vi "CH_LM App History.vi"(0 "Data":T1[](array[typedef]) {"Histogram"."X Values" format="%0.2f"; "Statistics"."Std. Dev." format="%#_4p"; "Statistics"."Max" format="%#_4p"; "Statistics"."Min" format="%#_4p"; "Statistics"."Mean" format="%#_4p"; "Data Cluster"."Flags" format="%.0b"; "Data Cluster"."Unit ID" format="%.0b"; "Data Cluster"."Quad Distance"."Y" format="%#.1f"; "Data Cluster"."Quad Distance"."X" format="%#.1f"; "Data Cluster"."Value" format="%#.7e"; "LabMax Device List Element"."Probe Diameter" format="%#.2g"}, 1 "Point(s)":i32, 2 "Sample Collection":enum32{"Fixed", "Continuous"}(ring), 3 "Sample Size":i32, 5 "Samples":i32, 7 "Point(s) Array":u32[](array[numeric]) min=1 max=20000, 9 "Points":i32, 11 "History in":T4[](array[typedef]) {"Stat. Min." format="%^#_7e"; "Stat. Max." format="%^#_7e"; "Maximum" format="%^#_7e"; "Live" format="%^#_7e"; "Value" format="%^#_7e"}, 12 "NofBins":i32, 13 "initialize Stat":bool, 14 "init Live Array":bool[](array[boolean])) -> (4 "Trend Data":T1[](array[typedef]) {"Histogram"."X Values" format="%0.2f"; "Statistics"."Std. Dev." format="%#_4p"; "Statistics"."Max" format="%#_4p"; "Statistics"."Min" format="%#_4p"; "Statistics"."Mean" format="%#_4p"; "Data Cluster"."Flags" format="%.0b"; "Data Cluster"."Unit ID" format="%.0b"; "Data Cluster"."Quad Distance"."Y" format="%#.1f"; "Data Cluster"."Quad Distance"."X" format="%#.1f"; "Data Cluster"."Value" format="%#.7e"; "LabMax Device List Element"."Probe Diameter" format="%#.2g"}, 15 "History out":T4[](array[typedef]) {"Stat. Min." format="%^#_7e"; "Stat. Max." format="%^#_7e"; "Maximum" format="%^#_7e"; "Live" format="%^#_7e"; "Value" format="%^#_7e"})   [LabVIEW 2012, in "CH_LM App.lvlib"]
doc: "This VI is used to calculate staticical properties, histogram data and to update the history data arrays."
uses:
  CH_LM App.lvlib
  <vilib>/Analysis/NI_AALBase.lvlib
  <vilib>/ptbypt/NI_PtbyPt.lvlib
  <vilib>/Analysis/baseanly.llb/Mean (DBL).vi
  CH_LM App DeviceListElement.ctl
  CH_LM/CH_LM Streaming Data.ctl
  CH_LM.lvlib
  CH_LM App TrendingData.ctl
  CH_LM App HistoryData.ctl
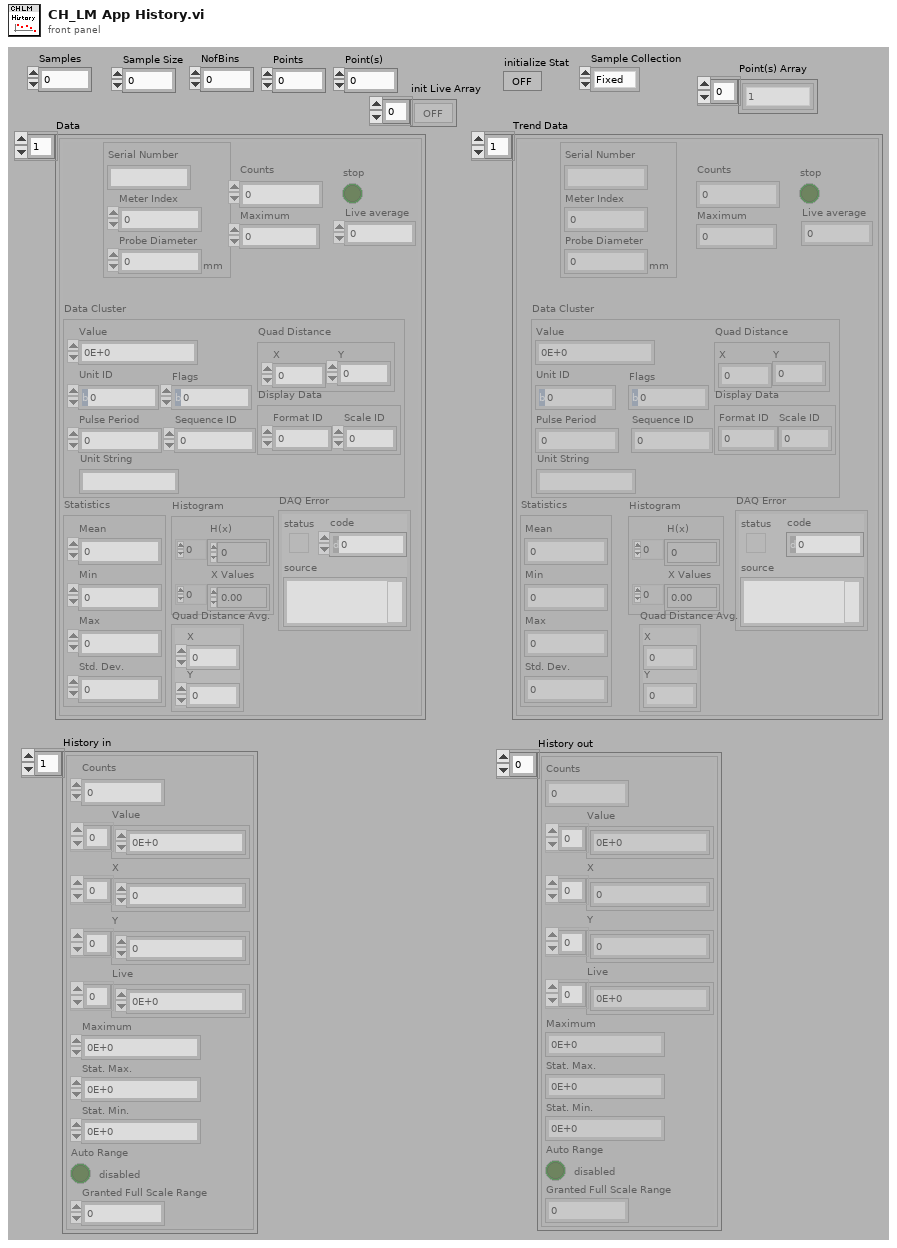
[diagram p1: front panel]
types:
  T1 = typedef "CH_LM App.lvlib/CH_LM App TrendingData.ctl" = cluster{"LabMax Device List Element":T2, "Data Cluster":T3, "Counts":i32, "Maximum":dbl, "Live average":dbl, "Statistics":cluster{"Mean":dbl, "Min":dbl, "Max":dbl, "Std. Dev.":dbl}, "Histogram":cluster{"H(x)":i32[], "X Values":dbl[]}, "DAQ Error":errorcluster, "stop":bool, "Quad Distance Avg.":cluster{"X":sgl, "Y":sgl}}
  T2 = typedef "CH_LM App.lvlib/CH_LM App DeviceListElement.ctl" = cluster{"Serial Number":string, "Meter Index":i32, "Probe Diameter":dbl[unit]}
  T3 = typedef "CH_LM.lvlib/CH_LM Streaming Data.ctl" = cluster{"Value":sgl, "Quad Distance":cluster{"X":sgl, "Y":sgl}, "Display Data":cluster{"Format ID":u8, "Scale ID":u8}, "Unit ID":u8, "Flags":u32, "Pulse Period":u32, "Sequence ID":u32, "Unit String":string}
  T4 = typedef "CH_LM App.lvlib/CH_LM App HistoryData.ctl" = cluster{"Counts":i32, "Value":sgl[], "X":sgl[], "Y":sgl[], "Live":sgl[], "Maximum":sgl, "Stat. Max.":sgl, "Stat. Min.":sgl, "Auto Range":bool, "Granted Full Scale Range":dbl}
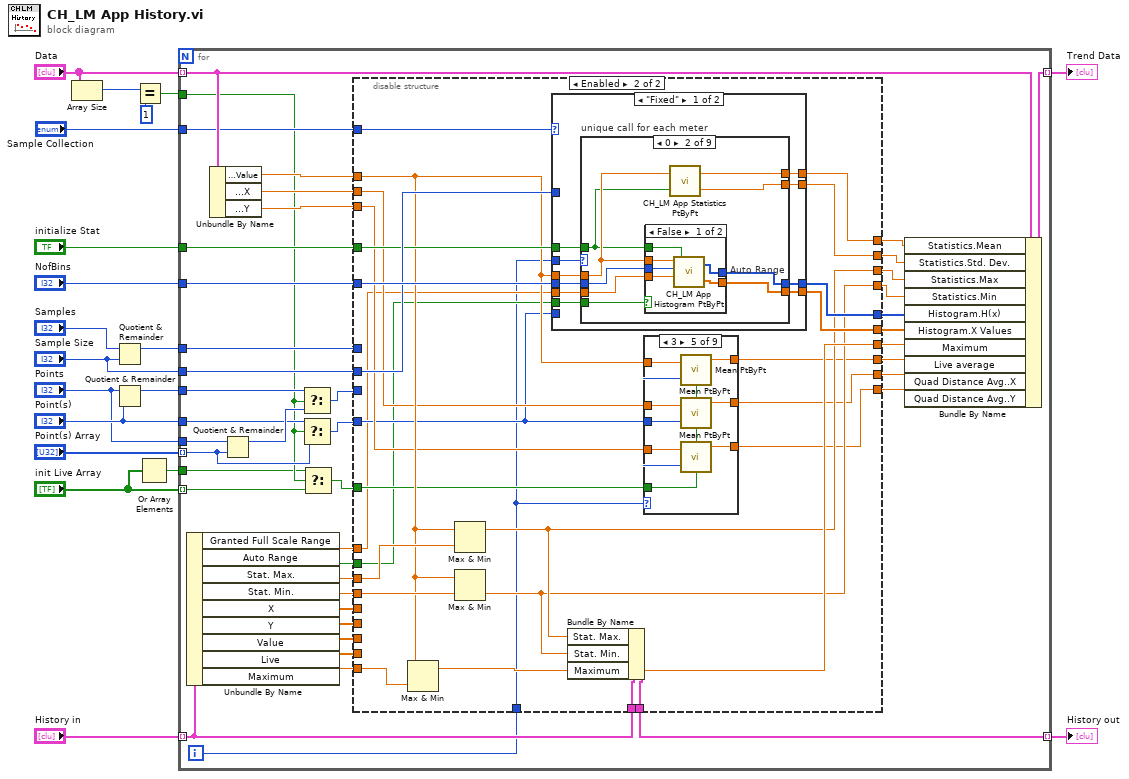
[diagram p0: block diagram]
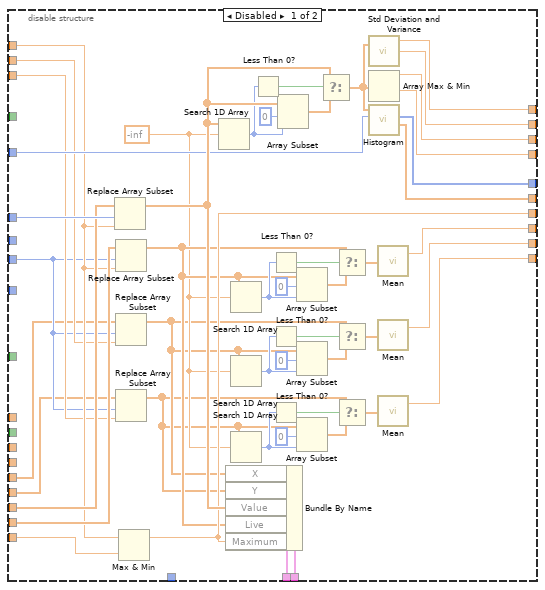
[diagram p2: hidden frame]
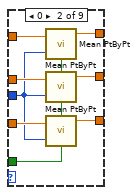
[diagram p4: hidden frame]
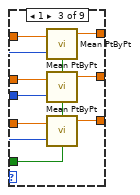
[diagram p5: hidden frame]
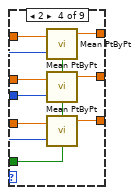
[diagram p6: hidden frame]
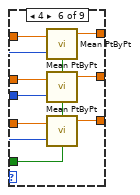
[diagram p7: hidden frame]
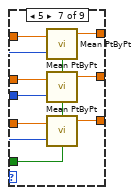
[diagram p8: hidden frame]
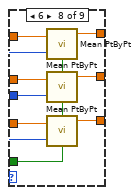
[diagram p9: hidden frame]
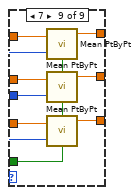
[diagram p10: hidden frame]
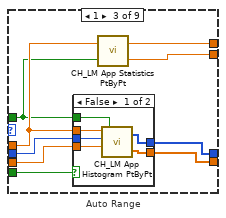
[diagram p13: hidden frame]
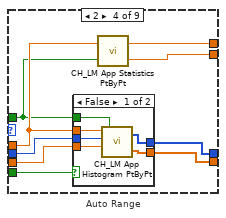
[diagram p15: hidden frame]
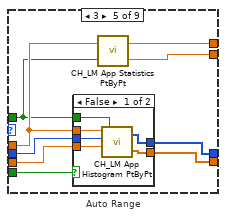
[diagram p17: hidden frame]
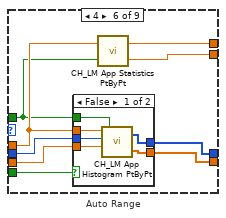
[diagram p19: hidden frame]
diagram:
  n1 = Array Size(array="Data") -> (size(s)=w5:i32)
  n2 = Quotient & Remainder(x="Samples", y="Sample Size") -> (x-y*floor(x/y)=w16:i32)  [unwired: 1 out]
  n3 = Quotient & Remainder(x="Points", y="Point(s)") -> (x-y*floor(x/y)=w13:i32)  [unwired: 1 out]
  n4 = Equal?(x=w5, y=1) -> (x = y?=w3:bool)
  n5 = Or Array Elements(Boolean array="init Live Array") -> (logical OR=w1:bool)
  n6 = for {
    tunnel: "Data" -> [w60] mode=indexing
    tunnel: "History in" -> [w51] mode=indexing
    tunnel: [w59] -> w18 mode=indexing
    tunnel: [w62] -> w17 mode=indexing
    tunnel: w16 -> [w61]
    tunnel: "NofBins" -> [w52]
    tunnel: w13 -> [w33]
    tunnel: "init Live Array" -> [w25] mode=indexing
    tunnel: "Sample Size" -> [w42]
    tunnel: "initialize Stat" -> [w39]
    tunnel: "Point(s)" -> [w30]
    tunnel: "Sample Collection" -> [w38]
    tunnel: "Point(s) Array" -> [w28] mode=indexing
    tunnel: "Points" -> [w34]
    tunnel: w3 -> [w27]
    tunnel: w1 -> [w24]
    i -> [w37]
    n7 = Unbundle By Name(w51) -> ("Granted Full Scale Range"=w36:dbl, "Auto Range"=w35:bool, "Stat. Max."=w41:sgl, "Stat. Min."=w40:sgl, "X"=w44:sgl[], "Y"=w43:sgl[], "Value"=w49:sgl[], "Live"=w50:sgl[], "Maximum"=w48:sgl)
    n8 = Unbundle By Name(w60) -> ("Data Cluster.Value"=w47:sgl, "Data Cluster.Quad Distance.X"=w46:sgl, "Data Cluster.Quad Distance.Y"=w45:sgl)
    n9 = Quotient & Remainder(x=w34, y=w28) -> (x-y*floor(x/y)=w31:u32)  [unwired: 1 out]
    n10 = Select(t=w33, s=w27, f=w31) -> (s? t:f=w32:u32)
    n11 = Select(t=w30, s=w27, f=w28) -> (s? t:f=w29:u32)
    n12 = Select(t=w24, s=w27, f=w25) -> (s? t:f=w26:bool)
    n13 = disable-structure shown="Enabled" {
      disable-tunnel: [w110 w133] -> w62
      disable-tunnel: w61 -> [w109 _]
      disable-tunnel: [w104 w137] -> w58
      disable-tunnel: [w103 w136] -> w57
      disable-tunnel: [w101 w127] -> w56
      disable-tunnel: [w100 w128] -> w55
      disable-tunnel: [w99 w112] -> w54
      disable-tunnel: [w98 w113] -> w53
      disable-tunnel: w52 -> [w97 w131]
      disable-tunnel: [w92 w124] -> w21
      disable-tunnel: w51 -> [w91 w134]
      disable-tunnel: w50 -> [w90 _]
      disable-tunnel: w49 -> [w89 _]
      disable-tunnel: w48 -> [w88 w135]
      disable-tunnel: w47 -> [w87 w123]
      disable-tunnel: [w86 w132] -> w20
      disable-tunnel: w46 -> [w72 w122]
      disable-tunnel: w45 -> [w71 w119]
      disable-tunnel: w32 -> [w70 _]
      disable-tunnel: w44 -> [w69 _]
      disable-tunnel: w43 -> [w68 _]
      disable-tunnel: [w66 w121] -> w22
      disable-tunnel: [w65 w118] -> w23
      disable-tunnel: w26 -> [_ w120]
      disable-tunnel: w42 -> [_ w126]
      disable-tunnel: w41 -> [_ w130]
      disable-tunnel: w40 -> [_ w129]
      disable-tunnel: w39 -> [_ w125]
      disable-tunnel: w29 -> [_ w117]
      disable-tunnel: w38 -> [_ w116]
      disable-tunnel: w37 -> [_ w111]
      disable-tunnel: w36 -> [_ w115]
      disable-tunnel: w35 -> [_ w114]
      frame Disabled {
        w67 = -inf ("element")
        n14 = Replace Array Subset(array=w89, new element=w87, index=w109) -> (w102:sgl[])
        n15 = Replace Array Subset(array=w90, new element=w87, index=w70) -> (w84:sgl[])
        n16 = Replace Array Subset(array=w69, new element=w72, index=w70) -> (w64:sgl[])
        n17 = Replace Array Subset(array=w68, new element=w71, index=w70) -> (w63:sgl[])
        n18 = Max & Min(x=w87, y=w88) -> (max(x,y)=w86:sgl)  [unwired: 1 out]
        n19 = Search 1D Array(1D array=w102, element=w67) -> (index of element=w85:i32)  [unwired: 1 in]
        n20 = Bundle By Name(cluster=w91, "X"=w64, "Y"=w63, "Value"=w102, "Live"=w84, "Maximum"=w86) -> (w110:T4)
        n21 = Search 1D Array(1D array=w84, element=w67) -> (index of element=w94:i32)  [unwired: 1 in]
        n22 = Search 1D Array(1D array=w64, element=w67) -> (index of element=w80:i32)  [unwired: 1 in]
        n23 = Search 1D Array(1D array=w63, element=w67) -> (index of element=w75:i32)  [unwired: 1 in]
        n24 = Less Than 0?(x=w85) -> (x < 0?=w106:bool)
        n25 = Less Than 0?(x=w94) -> (x < 0?=w95:bool)
        n26 = Less Than 0?(x=w80) -> (x < 0?=w79:bool)
        n27 = Less Than 0?(x=w75) -> (x < 0?=w76:bool)
        n28 = Array Subset(array=w102, index=0, length=w85) -> (w107:sgl[])
        n29 = Array Subset(array=w84, index=0, length=w94) -> (w83:sgl[])
        n30 = Array Subset(array=w64, index=0, length=w80) -> (w82:sgl[])
        n31 = Array Subset(array=w63, index=0, length=w75) -> (w73:sgl[])
        n32 = Select(t=w102, s=w106, f=w107) -> (s? t:f=w108:sgl[])
        n33 = Select(t=w84, s=w95, f=w83) -> (s? t:f=w96:sgl[])
        n34 = Select(t=w64, s=w79, f=w82) -> (s? t:f=w78:sgl[])
        n35 = Select(t=w63, s=w76, f=w73) -> (s? t:f=w77:sgl[])
        n36 = call <vilib>:"Std Deviation and Variance.vi"("X"=w108) -> ("mean"=w98:dbl, "standard deviation"=w99:dbl)  [unwired: 1 in, 1 out]
        n37 = Array Max & Min(array=w108) -> (max value=w100:sgl, min value=w101:sgl)  [unwired: 2 out]
        n38 = call <vilib>:"Histogram.vi"("intervals"=w97, "X"=w108) -> ("X Values"=w103:dbl[], "Histogram: h(x)"=w104:i32[])  [unwired: 6 in, 2 out]
        n39 = call-poly <vilib>:"Mean.vi"("X"=w96) -> ("mean"=w92:dbl)  [unwired: 1 out]
        n40 = call-poly <vilib>:"Mean.vi"("X"=w78) -> ("mean"=w66:dbl)  [unwired: 1 out]
        n41 = call-poly <vilib>:"Mean.vi"("X"=w77) -> ("mean"=w65:dbl)  [unwired: 1 out]
      }
      frame Enabled {
        n42 = Max & Min(x=w123, y=w135) -> (max(x,y)=w132:sgl)  [unwired: 1 out]
        n43 = Max & Min(x=w123, y=w130) -> (max(x,y)=w128:sgl)  [unwired: 1 out]
        n44 = Max & Min(x=w123, y=w129) -> (min(x,y)=w127:sgl)  [unwired: 1 out]
        n45 = case shown="\"Fixed\"" w116 {
          tunnel: [w208 w337] -> w137
          tunnel: [w207 w336] -> w136
          tunnel: [w210 w333] -> w112
          tunnel: [w211 w334] -> w113
          tunnel: w131 -> [w206 w339]
          tunnel: w126 -> [_ w338]
          tunnel: w125 -> [w205 w335]
          tunnel: w123 -> [w209 w340]
          tunnel: w117 -> [_ _]
          tunnel: w111 -> [w204 w332]
          tunnel: w115 -> [w203 _]
          tunnel: w114 -> [w202 _]
          frame "Fixed" {
            n46 = case "unique call for each meter" shown="0" w204 {
              tunnel: [_ w220 w235 w250 w265 w280 w295 w310 w325] -> w211
              tunnel: [_ w219 w234 w249 w264 w279 w294 w309 w324] -> w210
              tunnel: w209 -> [_ w218 w233 w248 w263 w278 w293 w308 w323]
              tunnel: [_ w217 w232 w247 w262 w277 w292 w307 w322] -> w208
              tunnel: [_ w216 w231 w246 w261 w276 w291 w306 w321] -> w207
              tunnel: w206 -> [_ w215 w230 w245 w260 w275 w290 w305 w320]
              tunnel: w205 -> [_ w214 w229 w244 w259 w274 w289 w304 w319]
              tunnel: w203 -> [_ w213 w228 w243 w258 w273 w288 w303 w318]
              tunnel: w202 -> [_ w212 w227 w242 w257 w272 w287 w302 w317]
              frame Default {
              }
              frame 0 {
                n47 = case "Auto Range" shown="False" w212 {
                  tunnel: w218 -> [w226 _]
                  tunnel: [w225 _] -> w217
                  tunnel: [w224 _] -> w216
                  tunnel: w215 -> [w223 _]
                  tunnel: w214 -> [w222 _]
                  tunnel: w213 -> [w221 _]
                  frame False {
                    n48 = call "CH_LM App Histogram PtByPt.vi"("initialize"=w222, "Range"=w221, "intervals"=w223, "x"=w226) -> ("X Values"=w224:dbl[], "Histogram: h(x)"=w225:i32[])
                  }
                  frame True {
                  }
                }
                n49 = call "CH_LM App Statistics PtByPt.vi"("initialize"=w214, "x"=w218) -> ("standard deviation"=w219:dbl, "mean"=w220:dbl)
              }
              frame 1 {
                n50 = case "Auto Range" shown="False" w227 {
                  tunnel: w233 -> [w241 _]
                  tunnel: [w240 _] -> w232
                  tunnel: [w239 _] -> w231
                  tunnel: w230 -> [w238 _]
                  tunnel: w229 -> [w237 _]
                  tunnel: w228 -> [w236 _]
                  frame False {
                    n51 = call "CH_LM App Histogram PtByPt.vi"("initialize"=w237, "Range"=w236, "intervals"=w238, "x"=w241) -> ("X Values"=w239:dbl[], "Histogram: h(x)"=w240:i32[])
                  }
                  frame True {
                  }
                }
                n52 = call "CH_LM App Statistics PtByPt.vi"("initialize"=w229, "x"=w233) -> ("standard deviation"=w234:dbl, "mean"=w235:dbl)
              }
              frame 2 {
                n53 = case "Auto Range" shown="False" w242 {
                  tunnel: w248 -> [w256 _]
                  tunnel: [w255 _] -> w247
                  tunnel: [w254 _] -> w246
                  tunnel: w245 -> [w253 _]
                  tunnel: w244 -> [w252 _]
                  tunnel: w243 -> [w251 _]
                  frame False {
                    n54 = call "CH_LM App Histogram PtByPt.vi"("initialize"=w252, "Range"=w251, "intervals"=w253, "x"=w256) -> ("X Values"=w254:dbl[], "Histogram: h(x)"=w255:i32[])
                  }
                  frame True {
                  }
                }
                n55 = call "CH_LM App Statistics PtByPt.vi"("initialize"=w244, "x"=w248) -> ("standard deviation"=w249:dbl, "mean"=w250:dbl)
              }
              frame 3 {
                n56 = case "Auto Range" shown="False" w257 {
                  tunnel: w263 -> [w271 _]
                  tunnel: [w270 _] -> w262
                  tunnel: [w269 _] -> w261
                  tunnel: w260 -> [w268 _]
                  tunnel: w259 -> [w267 _]
                  tunnel: w258 -> [w266 _]
                  frame False {
                    n57 = call "CH_LM App Histogram PtByPt.vi"("initialize"=w267, "Range"=w266, "intervals"=w268, "x"=w271) -> ("X Values"=w269:dbl[], "Histogram: h(x)"=w270:i32[])
                  }
                  frame True {
                  }
                }
                n58 = call "CH_LM App Statistics PtByPt.vi"("initialize"=w259, "x"=w263) -> ("standard deviation"=w264:dbl, "mean"=w265:dbl)
              }
              frame 4 {
                n59 = case "Auto Range" shown="False" w272 {
                  tunnel: w278 -> [w286 _]
                  tunnel: [w285 _] -> w277
                  tunnel: [w284 _] -> w276
                  tunnel: w275 -> [w283 _]
                  tunnel: w274 -> [w282 _]
                  tunnel: w273 -> [w281 _]
                  frame False {
                    n60 = call "CH_LM App Histogram PtByPt.vi"("initialize"=w282, "Range"=w281, "intervals"=w283, "x"=w286) -> ("X Values"=w284:dbl[], "Histogram: h(x)"=w285:i32[])
                  }
                  frame True {
                  }
                }
                n61 = call "CH_LM App Statistics PtByPt.vi"("initialize"=w274, "x"=w278) -> ("standard deviation"=w279:dbl, "mean"=w280:dbl)
              }
              frame 5 {
                n62 = case "Auto Range" shown="False" w287 {
                  tunnel: w293 -> [w301 _]
                  tunnel: [w300 _] -> w292
                  tunnel: [w299 _] -> w291
                  tunnel: w290 -> [w298 _]
                  tunnel: w289 -> [w297 _]
                  tunnel: w288 -> [w296 _]
                  frame False {
                    n63 = call "CH_LM App Histogram PtByPt.vi"("initialize"=w297, "Range"=w296, "intervals"=w298, "x"=w301) -> ("X Values"=w299:dbl[], "Histogram: h(x)"=w300:i32[])
                  }
                  frame True {
                  }
                }
                n64 = call "CH_LM App Statistics PtByPt.vi"("initialize"=w289, "x"=w293) -> ("standard deviation"=w294:dbl, "mean"=w295:dbl)
              }
              frame 6 {
                n65 = case "Auto Range" shown="False" w302 {
                  tunnel: w308 -> [w316 _]
                  tunnel: [w315 _] -> w307
                  tunnel: [w314 _] -> w306
                  tunnel: w305 -> [w313 _]
                  tunnel: w304 -> [w312 _]
                  tunnel: w303 -> [w311 _]
                  frame False {
                    n66 = call "CH_LM App Histogram PtByPt.vi"("initialize"=w312, "Range"=w311, "intervals"=w313, "x"=w316) -> ("X Values"=w314:dbl[], "Histogram: h(x)"=w315:i32[])
                  }
                  frame True {
                  }
                }
                n67 = call "CH_LM App Statistics PtByPt.vi"("initialize"=w304, "x"=w308) -> ("standard deviation"=w309:dbl, "mean"=w310:dbl)
              }
              frame 7 {
                n68 = case "Auto Range" shown="False" w317 {
                  tunnel: w323 -> [w331 _]
                  tunnel: [w330 _] -> w322
                  tunnel: [w329 _] -> w321
                  tunnel: w320 -> [w328 _]
                  tunnel: w319 -> [w327 _]
                  tunnel: w318 -> [w326 _]
                  frame False {
                    n69 = call "CH_LM App Histogram PtByPt.vi"("initialize"=w327, "Range"=w326, "intervals"=w328, "x"=w331) -> ("X Values"=w329:dbl[], "Histogram: h(x)"=w330:i32[])
                  }
                  frame True {
                  }
                }
                n70 = call "CH_LM App Statistics PtByPt.vi"("initialize"=w319, "x"=w323) -> ("standard deviation"=w324:dbl, "mean"=w325:dbl)
              }
            }
          }
          frame "Continuous", Default {
            n71 = case "unique call for each meter" shown="2" w332 {
              tunnel: w340 -> [_ w348 w356 w364 w372 w380 w388 w396 w404]
              tunnel: w339 -> [_ w347 w355 w363 w371 w379 w387 w395 w403]
              tunnel: w338 -> [_ w346 w354 w362 w370 w378 w386 w394 w402]
              tunnel: [_ w345 w353 w361 w369 w377 w385 w393 w401] -> w337
              tunnel: [_ w344 w352 w360 w368 w376 w384 w392 w400] -> w336
              tunnel: w335 -> [_ w343 w351 w359 w367 w375 w383 w391 w399]
              tunnel: [_ w342 w350 w358 w366 w374 w382 w390 w398] -> w334
              tunnel: [_ w341 w349 w357 w365 w373 w381 w389 w397] -> w333
              frame Default {
              }
              frame 0 {
                n72 = call <vilib>:"Standard Deviation PtByPt.vi"("x"=w348, "sample length"=w346, "initialize"=w343) -> ("standard deviation"=w341:dbl, "mean"=w342:dbl)  [unwired: 1 out]
                n73 = call <vilib>:"Histogram PtByPt.vi"("initialize"=w343, "sample length"=w346, "intervals"=w347, "x"=w348) -> ("X Values"=w344:dbl[], "Histogram: h(x)"=w345:i32[])  [unwired: 6 out]
              }
              frame 1 {
                n74 = call <vilib>:"Standard Deviation PtByPt.vi"("x"=w356, "sample length"=w354, "initialize"=w351) -> ("standard deviation"=w349:dbl, "mean"=w350:dbl)  [unwired: 1 out]
                n75 = call <vilib>:"Histogram PtByPt.vi"("initialize"=w351, "sample length"=w354, "intervals"=w355, "x"=w356) -> ("X Values"=w352:dbl[], "Histogram: h(x)"=w353:i32[])  [unwired: 6 out]
              }
              frame 2 {
                n76 = call <vilib>:"Standard Deviation PtByPt.vi"("x"=w364, "sample length"=w362, "initialize"=w359) -> ("standard deviation"=w357:dbl, "mean"=w358:dbl)  [unwired: 1 out]
                n77 = call <vilib>:"Histogram PtByPt.vi"("initialize"=w359, "sample length"=w362, "intervals"=w363, "x"=w364) -> ("X Values"=w360:dbl[], "Histogram: h(x)"=w361:i32[])  [unwired: 6 out]
              }
              frame 3 {
                n78 = call <vilib>:"Standard Deviation PtByPt.vi"("x"=w372, "sample length"=w370, "initialize"=w367) -> ("standard deviation"=w365:dbl, "mean"=w366:dbl)  [unwired: 1 out]
                n79 = call <vilib>:"Histogram PtByPt.vi"("initialize"=w367, "sample length"=w370, "intervals"=w371, "x"=w372) -> ("X Values"=w368:dbl[], "Histogram: h(x)"=w369:i32[])  [unwired: 6 out]
              }
              frame 4 {
                n80 = call <vilib>:"Standard Deviation PtByPt.vi"("x"=w380, "sample length"=w378, "initialize"=w375) -> ("standard deviation"=w373:dbl, "mean"=w374:dbl)  [unwired: 1 out]
                n81 = call <vilib>:"Histogram PtByPt.vi"("initialize"=w375, "sample length"=w378, "intervals"=w379, "x"=w380) -> ("X Values"=w376:dbl[], "Histogram: h(x)"=w377:i32[])  [unwired: 6 out]
              }
              frame 5 {
                n82 = call <vilib>:"Standard Deviation PtByPt.vi"("x"=w388, "sample length"=w386, "initialize"=w383) -> ("standard deviation"=w381:dbl, "mean"=w382:dbl)  [unwired: 1 out]
                n83 = call <vilib>:"Histogram PtByPt.vi"("initialize"=w383, "sample length"=w386, "intervals"=w387, "x"=w388) -> ("X Values"=w384:dbl[], "Histogram: h(x)"=w385:i32[])  [unwired: 6 out]
              }
              frame 6 {
                n84 = call <vilib>:"Standard Deviation PtByPt.vi"("x"=w396, "sample length"=w394, "initialize"=w391) -> ("standard deviation"=w389:dbl, "mean"=w390:dbl)  [unwired: 1 out]
                n85 = call <vilib>:"Histogram PtByPt.vi"("initialize"=w391, "sample length"=w394, "intervals"=w395, "x"=w396) -> ("X Values"=w392:dbl[], "Histogram: h(x)"=w393:i32[])  [unwired: 6 out]
              }
              frame 7 {
                n86 = call <vilib>:"Standard Deviation PtByPt.vi"("x"=w404, "sample length"=w402, "initialize"=w399) -> ("standard deviation"=w397:dbl, "mean"=w398:dbl)  [unwired: 1 out]
                n87 = call <vilib>:"Histogram PtByPt.vi"("initialize"=w399, "sample length"=w402, "intervals"=w403, "x"=w404) -> ("X Values"=w400:dbl[], "Histogram: h(x)"=w401:i32[])  [unwired: 6 out]
              }
            }
          }
        }
        n88 = Bundle By Name(cluster=w134, "Stat. Max."=w128, "Stat. Min."=w127, "Maximum"=w132) -> (w133:T4)
        n89 = case shown="3" w111 {
          tunnel: [_ w145 w153 w161 w169 w177 w185 w193 w201] -> w124
          tunnel: w123 -> [_ w144 w152 w160 w168 w176 w184 w192 w200]
          tunnel: w122 -> [_ w143 w151 w159 w167 w175 w183 w191 w199]
          tunnel: [_ w142 w150 w158 w166 w174 w182 w190 w198] -> w121
          tunnel: w120 -> [_ w141 w149 w157 w165 w173 w181 w189 w197]
          tunnel: w119 -> [_ w140 w148 w156 w164 w172 w180 w188 w196]
          tunnel: [_ w139 w147 w155 w163 w171 w179 w187 w195] -> w118
          tunnel: w117 -> [_ w138 w146 w154 w162 w170 w178 w186 w194]
          frame Default {
          }
          frame 0 {
            n90 = call <vilib>:"Mean PtByPt.vi"("x"=w144, "sample length"=w138, "initialize"=w141) -> ("mean"=w145:dbl)  [unwired: 2 out]
            n91 = call <vilib>:"Mean PtByPt.vi"("x"=w143, "sample length"=w138, "initialize"=w141) -> ("mean"=w142:dbl)  [unwired: 2 out]
            n92 = call <vilib>:"Mean PtByPt.vi"("x"=w140, "sample length"=w138, "initialize"=w141) -> ("mean"=w139:dbl)  [unwired: 2 out]
          }
          frame 1 {
            n93 = call <vilib>:"Mean PtByPt.vi"("x"=w152, "sample length"=w146, "initialize"=w149) -> ("mean"=w153:dbl)  [unwired: 2 out]
            n94 = call <vilib>:"Mean PtByPt.vi"("x"=w151, "sample length"=w146, "initialize"=w149) -> ("mean"=w150:dbl)  [unwired: 2 out]
            n95 = call <vilib>:"Mean PtByPt.vi"("x"=w148, "sample length"=w146, "initialize"=w149) -> ("mean"=w147:dbl)  [unwired: 2 out]
          }
          frame 2 {
            n96 = call <vilib>:"Mean PtByPt.vi"("x"=w160, "sample length"=w154, "initialize"=w157) -> ("mean"=w161:dbl)  [unwired: 2 out]
            n97 = call <vilib>:"Mean PtByPt.vi"("x"=w159, "sample length"=w154, "initialize"=w157) -> ("mean"=w158:dbl)  [unwired: 2 out]
            n98 = call <vilib>:"Mean PtByPt.vi"("x"=w156, "sample length"=w154, "initialize"=w157) -> ("mean"=w155:dbl)  [unwired: 2 out]
          }
          frame 3 {
            n99 = call <vilib>:"Mean PtByPt.vi"("x"=w168, "sample length"=w162, "initialize"=w165) -> ("mean"=w169:dbl)  [unwired: 2 out]
            n100 = call <vilib>:"Mean PtByPt.vi"("x"=w167, "sample length"=w162, "initialize"=w165) -> ("mean"=w166:dbl)  [unwired: 2 out]
            n101 = call <vilib>:"Mean PtByPt.vi"("x"=w164, "sample length"=w162, "initialize"=w165) -> ("mean"=w163:dbl)  [unwired: 2 out]
          }
          frame 4 {
            n102 = call <vilib>:"Mean PtByPt.vi"("x"=w176, "sample length"=w170, "initialize"=w173) -> ("mean"=w177:dbl)  [unwired: 2 out]
            n103 = call <vilib>:"Mean PtByPt.vi"("x"=w175, "sample length"=w170, "initialize"=w173) -> ("mean"=w174:dbl)  [unwired: 2 out]
            n104 = call <vilib>:"Mean PtByPt.vi"("x"=w172, "sample length"=w170, "initialize"=w173) -> ("mean"=w171:dbl)  [unwired: 2 out]
          }
          frame 5 {
            n105 = call <vilib>:"Mean PtByPt.vi"("x"=w184, "sample length"=w178, "initialize"=w181) -> ("mean"=w185:dbl)  [unwired: 2 out]
            n106 = call <vilib>:"Mean PtByPt.vi"("x"=w183, "sample length"=w178, "initialize"=w181) -> ("mean"=w182:dbl)  [unwired: 2 out]
            n107 = call <vilib>:"Mean PtByPt.vi"("x"=w180, "sample length"=w178, "initialize"=w181) -> ("mean"=w179:dbl)  [unwired: 2 out]
          }
          frame 6 {
            n108 = call <vilib>:"Mean PtByPt.vi"("x"=w192, "sample length"=w186, "initialize"=w189) -> ("mean"=w193:dbl)  [unwired: 2 out]
            n109 = call <vilib>:"Mean PtByPt.vi"("x"=w191, "sample length"=w186, "initialize"=w189) -> ("mean"=w190:dbl)  [unwired: 2 out]
            n110 = call <vilib>:"Mean PtByPt.vi"("x"=w188, "sample length"=w186, "initialize"=w189) -> ("mean"=w187:dbl)  [unwired: 2 out]
          }
          frame 7 {
            n111 = call <vilib>:"Mean PtByPt.vi"("x"=w200, "sample length"=w194, "initialize"=w197) -> ("mean"=w201:dbl)  [unwired: 2 out]
            n112 = call <vilib>:"Mean PtByPt.vi"("x"=w199, "sample length"=w194, "initialize"=w197) -> ("mean"=w198:dbl)  [unwired: 2 out]
            n113 = call <vilib>:"Mean PtByPt.vi"("x"=w196, "sample length"=w194, "initialize"=w197) -> ("mean"=w195:dbl)  [unwired: 2 out]
          }
        }
      }
    }
    n114 = Bundle By Name(cluster=w60, "Statistics.Mean"=w53, "Statistics.Std. Dev."=w54, "Statistics.Max"=w55, "Statistics.Min"=w56, "Histogram.H(x)"=w58, "Histogram.X Values"=w57, "Maximum"=w20, "Live average"=w21, "Quad Distance Avg..X"=w22, "Quad Distance Avg..Y"=w23) -> (w59:T1)
  }
  "Trend Data" <- w18
  "History out" <- w17
